vi "IC_RestoreDevice.vi"(10 "filename":string, 11 ".NET Refnum in":refnum<k24>) -> (0 "error out":errorcluster, 2 "DeviceValid":bool, 3 ".NET Refnum out":refnum<k24>)   [LabVIEW 2013]
uses:
  TIS.Imaging.ICImagingControl34
  <vilib>/Utility/error.llb/DialogType.ctl
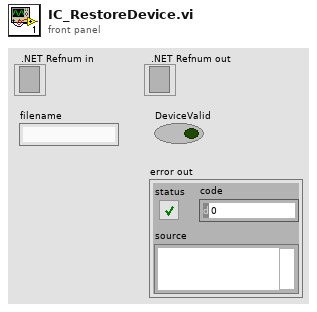
[diagram p1: front panel]
types:
  T1 = typedef "DialogType.ctl" = u16
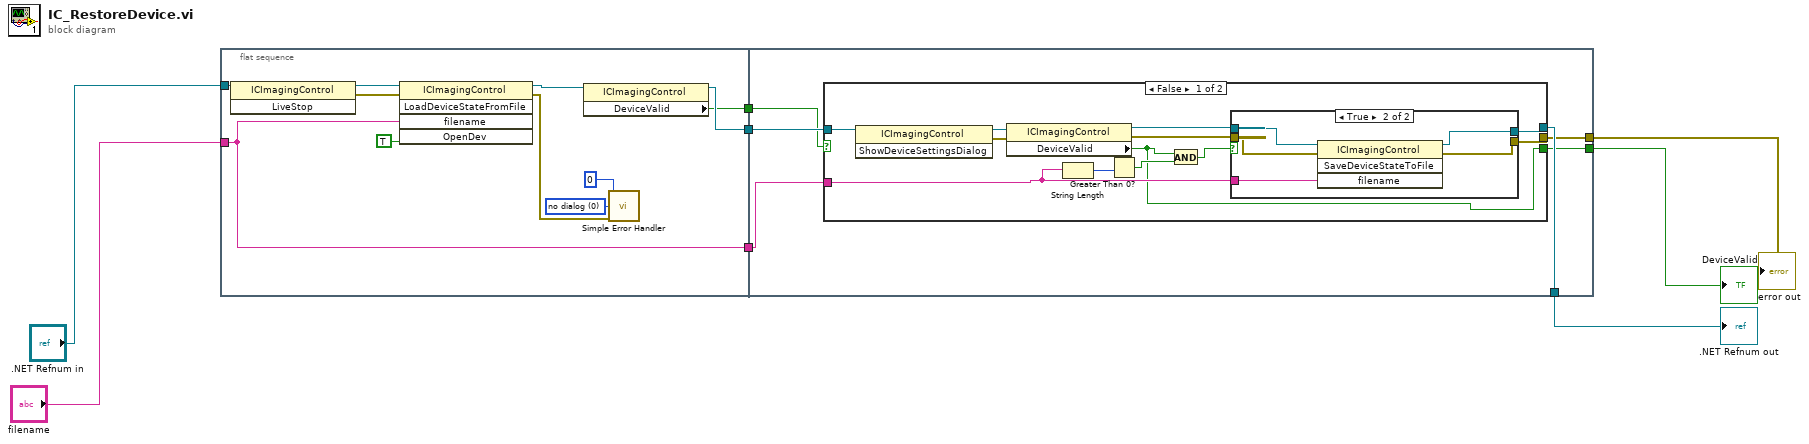
[diagram p0: block diagram]
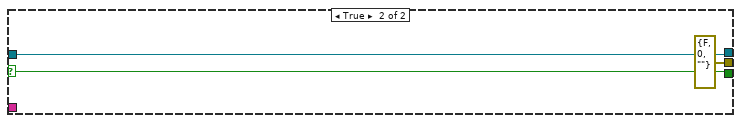
[diagram p3: hidden frame]
diagram:
  n1 = flat-sequence {
    tunnel: ".NET Refnum in" -> [w12]
    tunnel: "filename" -> [w9]
    tunnel: [w11] -> w8
    tunnel: [w10] -> w7
    tunnel: [w9] -> w6
    tunnel: w8 -> [w25]
    tunnel: w7 -> [w24]
    tunnel: w6 -> [w23]
    tunnel: [w22] -> w3
    tunnel: [w21] -> w4
    tunnel: [w20] -> w5
    frame #0 {
      w18 = T1 0 items=["no dialog", "OK message", "continue or stop message", "OK message + warnings", "continue/stop + warnings"] ("type of dialog (OK msg:1)")
      n2 = invoke class="ICImagingControl" method="LiveStop"(reference=w12) -> (reference out=w13:refnum<k24>, error out=w15:errorcluster)  [unwired: 2 in, 1 out]
      n3 = invoke class="ICImagingControl" method="LoadDeviceStateFromFile"(reference=w13, error in=w15, "filename"=w9, "OpenDev"=TRUE) -> (reference out=w16:refnum<k24>, error out=w19:errorcluster)  [unwired: 1 in, 3 out]
      n4 = property class="ICImagingControl"(reference=w16) -> (reference out=w11:refnum<k24>, "DeviceValid"=w10:bool)  [unwired: 1 in, 1 out]
      n5 = call <vilib>:"Simple Error Handler.vi"("error code (no error:0)"=0, "type of dialog (OK msg:1)"=w18, "error in (no error)"=w19) -> ()  [unwired: 2 in, 5 out]
    }
    frame #1 {
      n6 = case shown="False" w24 {
        selector: w24 -> [_ w47]
        tunnel: [w26 w47] -> w20
        tunnel: [w33 w46] -> w22
        tunnel: [w32 errorcluster {"status"=FALSE, "code"=0, "source"=""} ("error out")] -> w21
        tunnel: w25 -> [w31 w46]
        tunnel: w23 -> [w30 _]
        frame False {
          n7 = invoke class="ICImagingControl" method="ShowDeviceSettingsDialog"(reference=w31) -> (reference out=w37:refnum<k24>, error out=w36:errorcluster)  [unwired: 2 in, 1 out]
          n8 = property class="ICImagingControl"(reference=w37, error in=w36) -> (reference out=w34:refnum<k24>, error out=w35:errorcluster, "DeviceValid"=w26:bool)
          n9 = String Length(string=w30) -> (length=w29:i32)
          n10 = Greater Than 0?(x=w29) -> (x > 0?=w28:bool)
          n11 = And(x=w26, y=w28) -> (x .and. y?=w27:bool)
          n12 = case shown="True" w27 {
            tunnel: w35 -> [w38 w44]
            tunnel: w34 -> [w39 w43]
            tunnel: [w39 w42] -> w33
            tunnel: [w38 w41] -> w32
            tunnel: w30 -> [_ w40]
            frame False {
            }
            frame True {
              n13 = invoke class="ICImagingControl" method="SaveDeviceStateToFile"(reference=w43, error in=w44, "filename"=w40) -> (reference out=w42:refnum<k24>, error out=w41:errorcluster)  [unwired: 1 in, 2 out]
            }
          }
        }
        frame True {
        }
      }
    }
  }
  "DeviceValid" <- w5
  "error out" <- w4
  ".NET Refnum out" <- w3
